vi "Sector Analysis Module.vi"() -> (2 "State":T1)   [LabVIEW 2013]
uses:
  Sector Analysis Module Enum.ctl
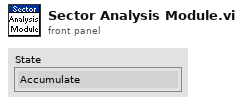
[diagram p1: front panel]
types:
  T1 = typedef "Sector Analysis Module Enum.ctl" = enum16{"Accumulate", "Analysis"}
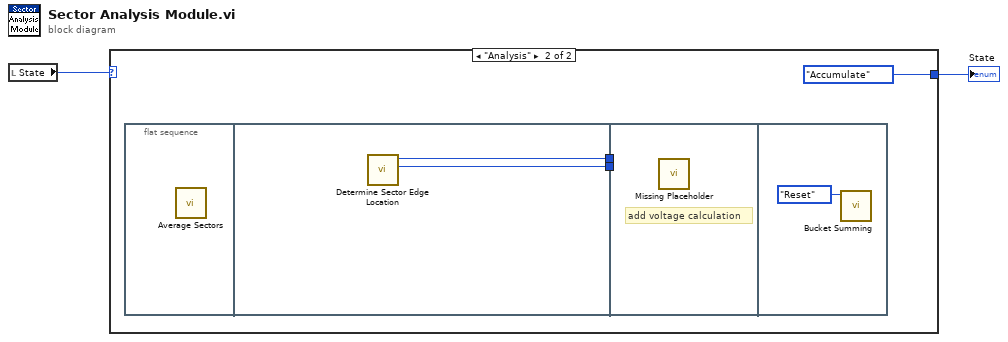
[diagram p0: block diagram]
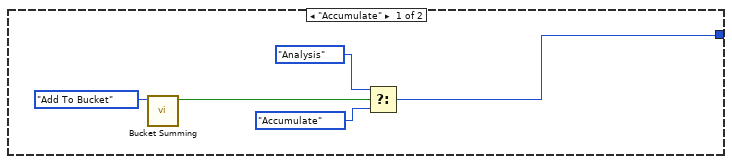
[diagram p2: hidden frame]
diagram:
  n1 = local read "State"() -> (w2:T1)
  n2 = case shown="\"Analysis\"" w2 {
    tunnel: [w3 Sector_Analysis_Module_Enum."Accumulate" ("State")] -> w1
    frame "Accumulate" {
      n3 = call "Bucket Summing.vi"("Bucket Summing State In"=enum16{"Reset", "Add To Bucket"}."Add To Bucket") -> ("Accumulation Complete?"=w6:bool)  [unwired: 10 in]
      n4 = Select(t=Sector_Analysis_Module_Enum."Analysis" ("State"), s=w6, f=Sector_Analysis_Module_Enum."Accumulate" ("State")) -> (s? t:f=w3:T1)
    }
    frame "Analysis" {
      n5 = flat-sequence {
        tunnel: [w12] -> w9
        tunnel: [w11] -> w8
        tunnel: w9 -> [_]
        tunnel: w8 -> [_]
        frame #0 {
          n6 = call "Average Sectors.vi"() -> ()  [unwired: 12 in]
        }
        frame #1 {
          n7 = call "Determine Sector Edge Location.vi"() -> ("Right Sector Edge"=w11:u8, "Left Sector Edge"=w12:u8)  [unwired: 10 in]
        }
        frame #2 {
          # "add voltage calculation"
          n8 = call "Missing Placeholder.vi"() -> ()  [unwired: 12 in]
        }
        frame #3 {
          n9 = call "Bucket Summing.vi"("Bucket Summing State In"=enum16{"Reset", "Add To Bucket"}."Reset") -> ()  [unwired: 10 in, 1 out]
        }
      }
    }
  }
  "State" <- w1
